vi "Normal Probability Plot.vi"(11 "Data array":dbl[](array[numeric]) format="%#.6g") -> (3 "Normal Probability Plot":cluster{"x":dbl, dbl}[](graph))   [LabVIEW 2023]
doc: "Computes the normal probability plot for the data."
uses:
  <vilib>/gmath/statdist.llb/Normal Inverse CDF.vi
  <vilib>/gmath/NI_Gmath.lvlib
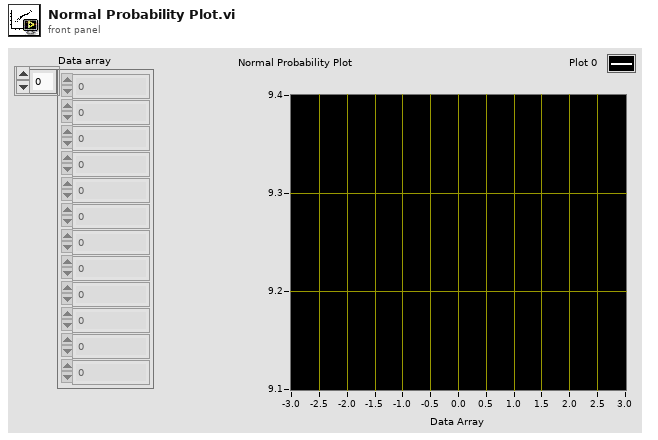
[diagram p1: front panel]
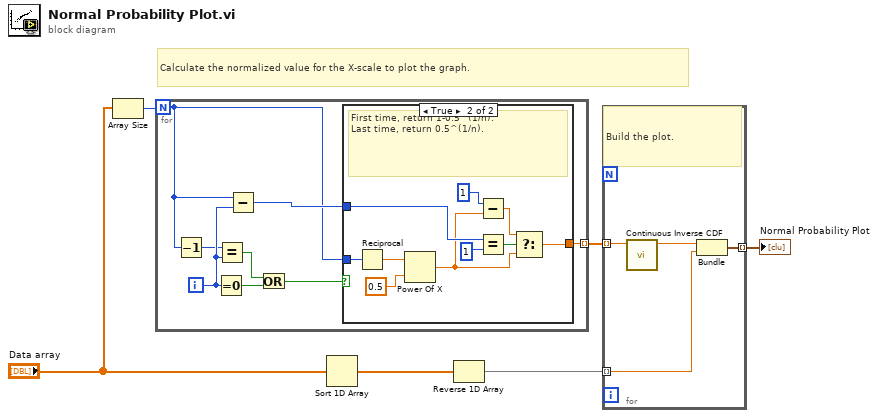
[diagram p0: block diagram]
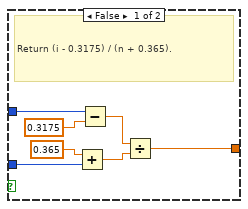
[diagram p2: hidden frame]
diagram:
  # "Calculate the normalized value for the X-scale to plot the graph."
  n1 = Array Size(array="Data array") -> (size(s)=w5:i32)
  n2 = for {
    N: w5 -> [w7]
    tunnel: [w8] -> w4 mode=indexing
    i -> [w13]
    n3 = Decrement(x=w7) -> (x-1=w9:i32)
    n4 = Equal To 0?(x=w13) -> (x = 0?=w12:bool)
    n5 = Equal?(x=w9, y=w13) -> (x = y?=w11:bool)
    n6 = Subtract(x=w7, y=w13) -> (x-y=w14:i32)
    n7 = Or(x=w11, y=w12) -> (x .or. y?=w10:bool)
    n8 = case shown="True" w10 {
      tunnel: w14 -> [w21 w29]
      tunnel: w7 -> [w19 w30]
      tunnel: [w16 w23] -> w8
      frame False {
        # "Return (i - 0.3175) / (n + 0.365)."
        n9 = Add(x=0.365, y=w19) -> (x+y=w17:dbl)
        n10 = Subtract(x=w21, y=0.3175) -> (x-y=w18:dbl)
        n11 = Divide(x=w18, y=w17) -> (x/y=w16:dbl)
      }
      frame True {
        # "First time, return 1-0.5^(1/n).\nLast time, return 0.5^(1/n)."
        n12 = Reciprocal(x=w30) -> (1/x=w31:dbl)
        n13 = Power Of X(1:0.5, 2:w31) -> (0:w26:dbl)
        n14 = Subtract(x=1, y=w26) -> (x-y=w24:dbl)
        n15 = Equal?(x=w29, y=1) -> (x = y?=w27:bool)
        n16 = Select(t=w24, s=w27, f=w26) -> (s? t:f=w23:dbl)
      }
    }
  }
  n17 = Sort 1D Array(array="Data array") -> (sorted array=w3:dbl[])
  n18 = Reverse 1D Array(array=w3) -> (reversed array=w2:dbl[])
  n19 = for {
    tunnel: w2 -> [w34] mode=indexing
    tunnel: [w35] -> w6 mode=indexing
    tunnel: w4 -> [w33] mode=indexing
    # "Build the plot."
    n20 = call-poly <vilib>:"Continuous Inverse CDF.vi"("cdf(x)"=w33) -> ("x"=w32:dbl)  [unwired: 9 in, 1 out]
    n21 = Bundle("x"=w32, w34) -> (w35:cluster{"x":dbl, dbl})  [unwired: 1 in]
  }
  "Normal Probability Plot" <- w6
